vi "CreateVirtualFolder.vi"(8 "error in (no error)":errorcluster, 11 "Project in":refnum<vi>) -> (0 "error out":errorcluster, 3 "VirtualFolderRef[]":refnum<vi>)   [LabVIEW 2021, in "Converter.lvlib"]
uses:
  Converter.lvlib
  Converter Reusables/Converter Reusables.lvlib
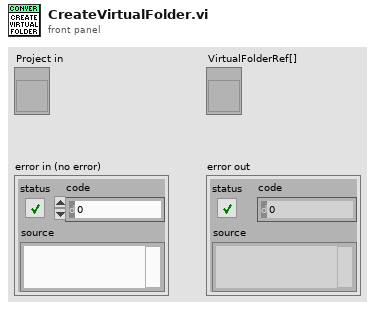
[diagram p1: front panel]
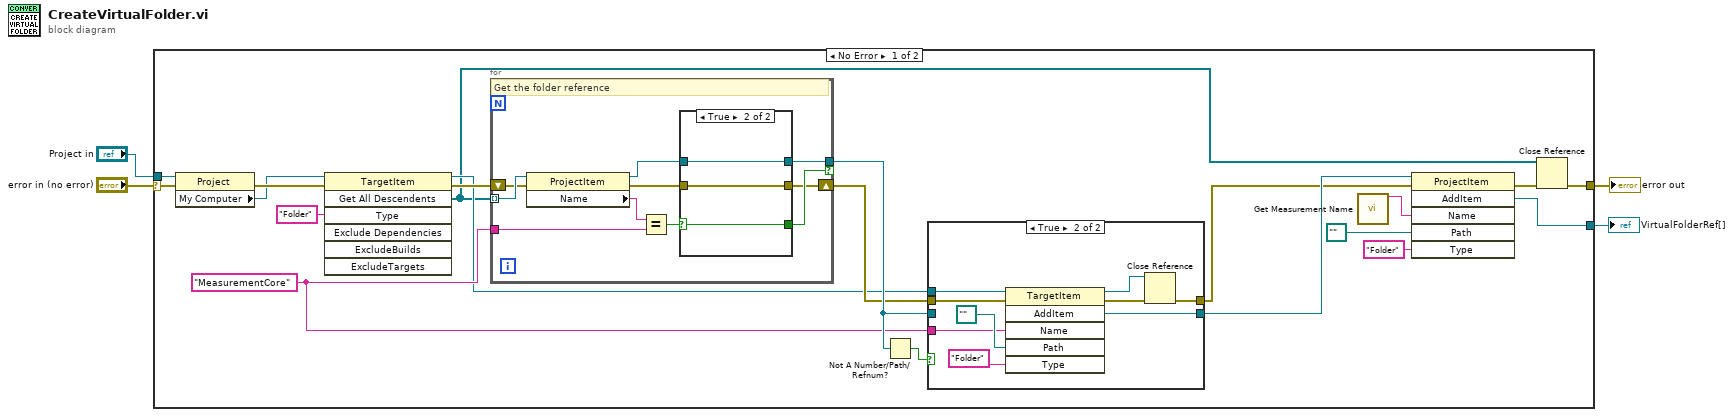
[diagram p0: block diagram]
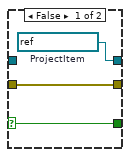
[diagram p2: hidden frame]
diagram:
  n1 = case shown="No Error" "error in (no error)" {
    selector: "error in (no error)" -> [w24 w52]
    tunnel: "Project in" -> [w22 _]
    tunnel: [w17 _] -> w2
    tunnel: [w16 w52] -> w1
    frame No Error {
      w11 = "MeasurementCore" ("Name")
      n2 = property class="Project"(reference=w22, error in=w24) -> (error out=w23:errorcluster, "My Computer"=w9:refnum<vi>)  [unwired: 1 out]
      n3 = invoke class="TargetItem" method="Get All Descendents"(reference=w9, error in=w23, "Type"="Folder") -> (reference out=w7:refnum<vi>, error out=w8:errorcluster, "All Descendents"=w5:refnum<vi>[])  [unwired: 4 in, 4 out]
      n4 = for {
        tunnel: w5 -> [w34] mode=indexing
        shift-right: [w25] -> w12
        shift-left: w8 -> [w31]
        tunnel: w11 -> [w29]
        tunnel: [w27] -> w13 if=w26
        # "Get the folder reference"
        n5 = property class="ProjectItem"(reference=w34, error in=w31) -> (reference out=w32:refnum<vi>, error out=w33:errorcluster, "Name"=w30:string)
        n6 = Equal?(x=w30, y=w29) -> (x = y?=w28:bool)
        n7 = case shown="True" w28 {
          selector: w28 -> [w36 w39]
          tunnel: w33 -> [w37 w38]
          tunnel: w32 -> [_ w40]
          tunnel: [w35 w40] -> w27
          tunnel: [w36 w39] -> w26
          tunnel: [w37 w38] -> w25
          frame False {
            w35 = refnum<vi> refnum  # ProjectItem
          }
          frame True {
          }
        }
      }
      n8 = Not A Number/Path/Refnum?(number/path/refnum=w13) -> (NaN/Path/Refnum?=w15:bool)
      n9 = case shown="True" w15 {
        tunnel: [w42 w47] -> w14
        tunnel: w13 -> [w42 _]
        tunnel: w12 -> [w41 w46]
        tunnel: w11 -> [_ w45]
        tunnel: [w41 w44] -> w6
        tunnel: w7 -> [_ w43]
        frame False {
        }
        frame True {
          n10 = invoke class="TargetItem" method="AddItem"(reference=w43, error in=w46, "Name"=w45, "Path"=path "", "Type"="Folder") -> (reference out=w50:refnum<vi>, error out=w51:errorcluster, "AddItem"=w47:refnum<vi>)  [unwired: 1 in, 3 out]
          n11 = Close Reference(reference=w50, error in (no error)=w51) -> (error out=w44:errorcluster)
        }
      }
      n12 = call "Get Measurement Name.vi"() -> ("Name Out"=w21:string)  [unwired: 14 in, 1 out]
      n13 = invoke class="ProjectItem" method="AddItem"(reference=w14, error in=w6, "Name"=w21, "Path"=path "", "Type"="Folder") -> (error out=w20:errorcluster, "AddItem"=w17:refnum<vi>)  [unwired: 1 in, 4 out]
      n14 = Close Reference(reference=w5, error in (no error)=w20) -> (error out=w16:errorcluster)
    }
    frame Error {
    }
  }
  "error out" <- w1
  "VirtualFolderRef[]" <- w2
